vi "Initialize.vi"   [LabVIEW 2017, in "nisyscfg.lvlib"]
doc: "<B>NOTE:</B> This VI has been replaced by the Initialize Session VI on the System Configuration palette.\n\nInitializes any system configuration VI to gather information from a specified target. You must use this VI to obtain a handle for a specified target that can be used in other System Configuration VIs."
uses:
  <vilib>/nisyscfg/nisyscfg.lvlib
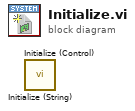
[diagram p0: block diagram]
diagram:
  n1 = call <vilib>:"Initialize (String).vi"() -> ()  [unwired: 9 in, 3 out]
  n2 = call <vilib>:"Initialize (Control).vi"() -> ()  [unwired: 9 in, 3 out]
